vi "Handle Command.vi"(8 "error in (no error)":errorcluster, 9 "Data":variant, 10 "Command":string, 11 "Example Instrument in":refnum<class "Instrument.LN2.lvclass">) -> (0 "error out":errorcluster, 1 "Processed Data":variant, 2 "Command":string, 3 "Example Instrument out":refnum<class "Instrument.LN2.lvclass">)   [LabVIEW 2019, in "Instrument.LN2.lvclass"]
uses:
  Instrument.LN2.lvclass
  Typedefs/Instrument.LN2.Commands--Enum.ctl
  Typedefs/Instrument.LN2.getAll--Cluster.ctl
  Instrument.LN2.lvclass/Instrument.LN2.ctl
  <userlib>/LevyLab/Instrument Framework/Instrument Types/VSource/Instrument.VSource.lvclass
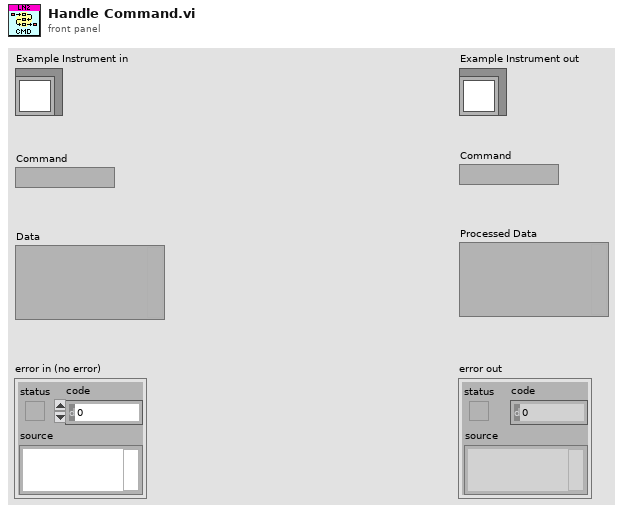
[diagram p1: front panel]
types:
  T1 = typedef "Instrument.LN2.lvclass/Instrument.LN2.Commands--Enum.ctl" = enum16{"Get weight"}
  T2 = typedef "Instrument.LN2.lvclass/Instrument.LN2.getAll--Cluster.ctl" = cluster{"Net Weight(lbs)":dbl, "Level":dbl, "Status":string}
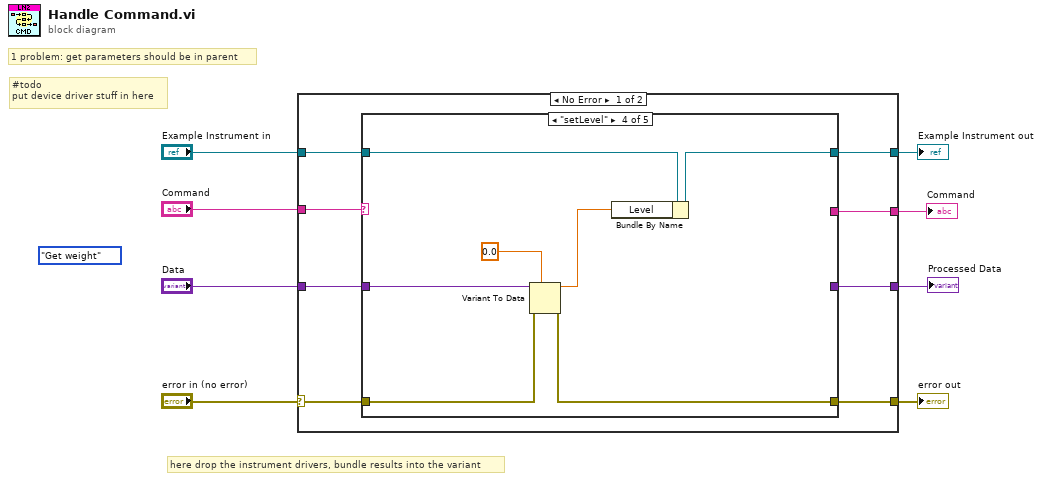
[diagram p0: block diagram]
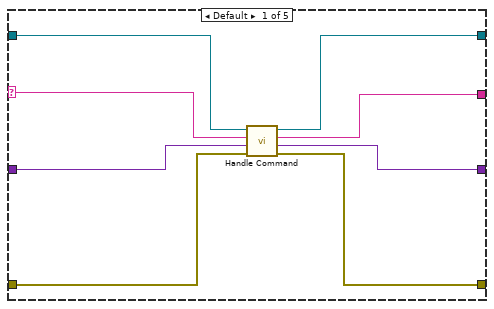
[diagram p2: hidden frame]
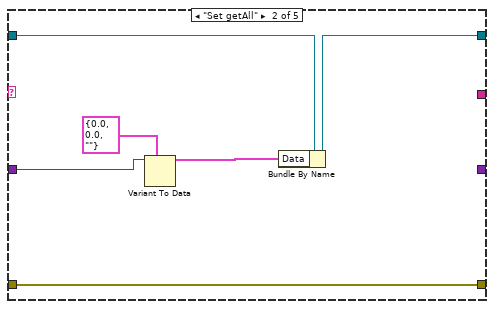
[diagram p3: hidden frame]
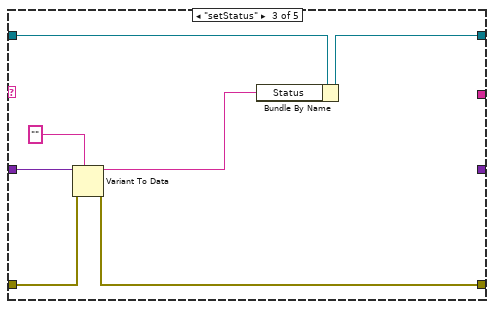
[diagram p4: hidden frame]
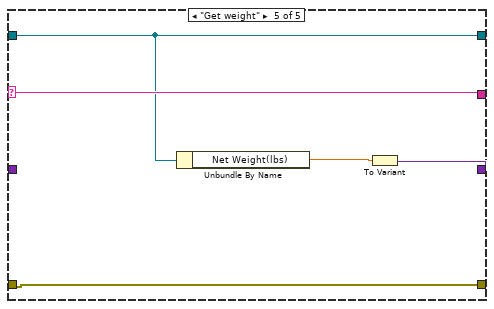
[diagram p5: hidden frame]
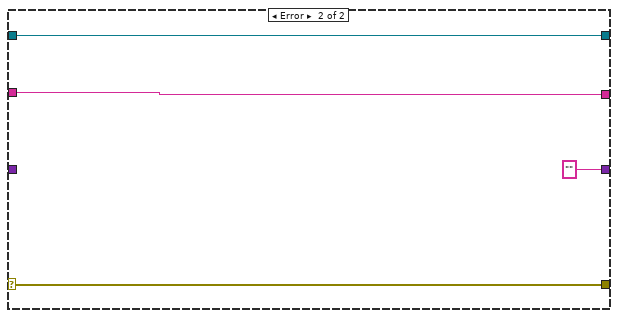
[diagram p6: hidden frame]
diagram:
  (unwired) Instrument.LN2.Commands--Enum."Get weight" ("Commands")
  # "here drop the instrument drivers, bundle results into the variant"
  # "1 problem: get parameters should be in parent"
  # "#todo\nput device driver stuff in here"
  n1 = case shown="No Error" "error in (no error)" {
    selector: "error in (no error)" -> [w12 w53]
    tunnel: [w10 w53] -> w7
    tunnel: [w14 w52] -> w6
    tunnel: "Example Instrument in" -> [w15 w52]
    tunnel: "Command" -> [w16 w50]
    tunnel: [w13 "" ("String")] -> w4
    tunnel: "Data" -> [w11 _]
    tunnel: [w9 w50] -> w2
    frame No Error {
      n2 = case shown="\"setLevel\"" w16 {
        selector: w16 -> [w24 _ _ _ w49]
        tunnel: w15 -> [w21 w28 w37 w44 w46]
        tunnel: [w18 w27 w36 w43 w46] -> w14
        tunnel: [w20 _ _ _ w47] -> w13
        tunnel: w12 -> [w22 w25 w32 w39 w48]
        tunnel: w11 -> [w23 w29 w35 w42 _]
        tunnel: [w19 w25 w31 w38 w48] -> w10
        tunnel: [w17 _ _ _ w49] -> w9
        frame Default {
          n3 = call-parent "Handle Command.vi"("error in (no error)"=w22, "Data"=w23, "Command"=w24, "Instrument in"=w21) -> ("error out"=w19:errorcluster, "Processed Data"=w20:variant, "Command"=w17:string, "Instrument out"=w18:refnum<class "Instrument.LN2.lvclass">)  [unwired: 4 in]
        }
        frame "Set getAll" {
          n4 = Variant To Data(type=T2 {"Net Weight(lbs)"=0.0, "Level"=0.0, "Status"=""} ("getAll"), Variant=w29) -> (data=w26:T2)  [unwired: 1 in, 1 out]
          n5 = Bundle By Name(cluster=w28, "Data"=w26) -> (w27:refnum<class "Instrument.LN2.lvclass">)
        }
        frame "setStatus" {
          n6 = Variant To Data(error in=w32, type="", Variant=w35) -> (data=w34:string, error out=w31:errorcluster)
          n7 = Bundle By Name(cluster=w37, "Status"=w34) -> (w36:refnum<class "Instrument.LN2.lvclass">)
        }
        frame "setLevel" {
          n8 = Variant To Data(error in=w39, type=0.0, Variant=w42) -> (data=w41:dbl, error out=w38:errorcluster)
          n9 = Bundle By Name(cluster=w44, "Level"=w41) -> (w43:refnum<class "Instrument.LN2.lvclass">)
        }
        frame "Get weight" {
          n10 = Unbundle By Name(w46) -> ("Net Weight(lbs)"=w45:dbl)
          n11 = To Variant(anything=w45) -> (Variant=w47:variant)
        }
      }
    }
    frame Error {
    }
  }
  "error out" <- w7
  "Example Instrument out" <- w6
  "Command" <- w2
  "Processed Data" <- w4
